vi "velodyne_parse.vi"(5 "Raw LiDAR data":string) -> (1 "Pased LIDAR Data":T1(array[cluster]), 3 "Timestamps":u32[](array[numeric]))   [LabVIEW 2019]
doc: "Parse UDP packet from Velodyne HDL."
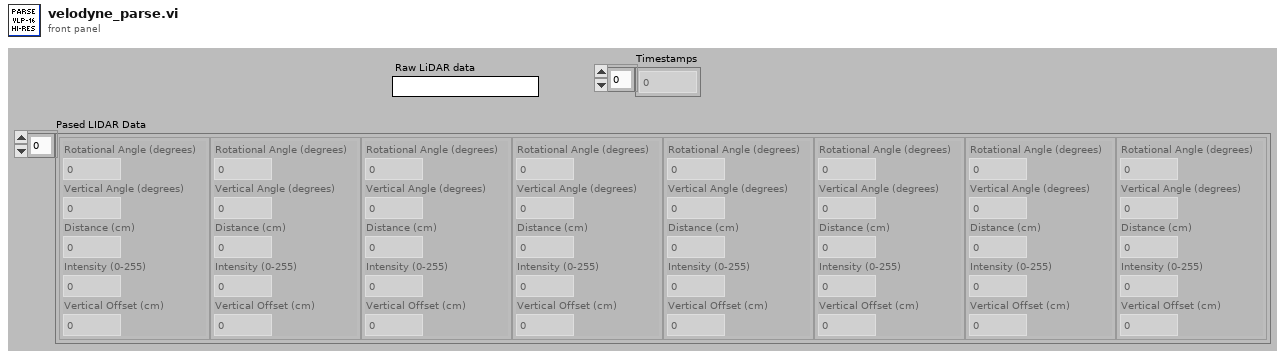
[diagram p1: front panel]
types:
  T1 = cluster{"Rotational Angle (degrees)":dbl, "Vertical Angle (degrees)":dbl, "Distance (cm)":dbl, "Intensity (0-255)":u8, "Vertical Offset (cm)":dbl}[]
  T2 = cluster{"Rotational Angle (degrees)":dbl, "Vertical Angle (degrees)":dbl, "Distance (cm)":dbl, "Intensity (0-255)":u8, "Vertical Offset (cm)":dbl}
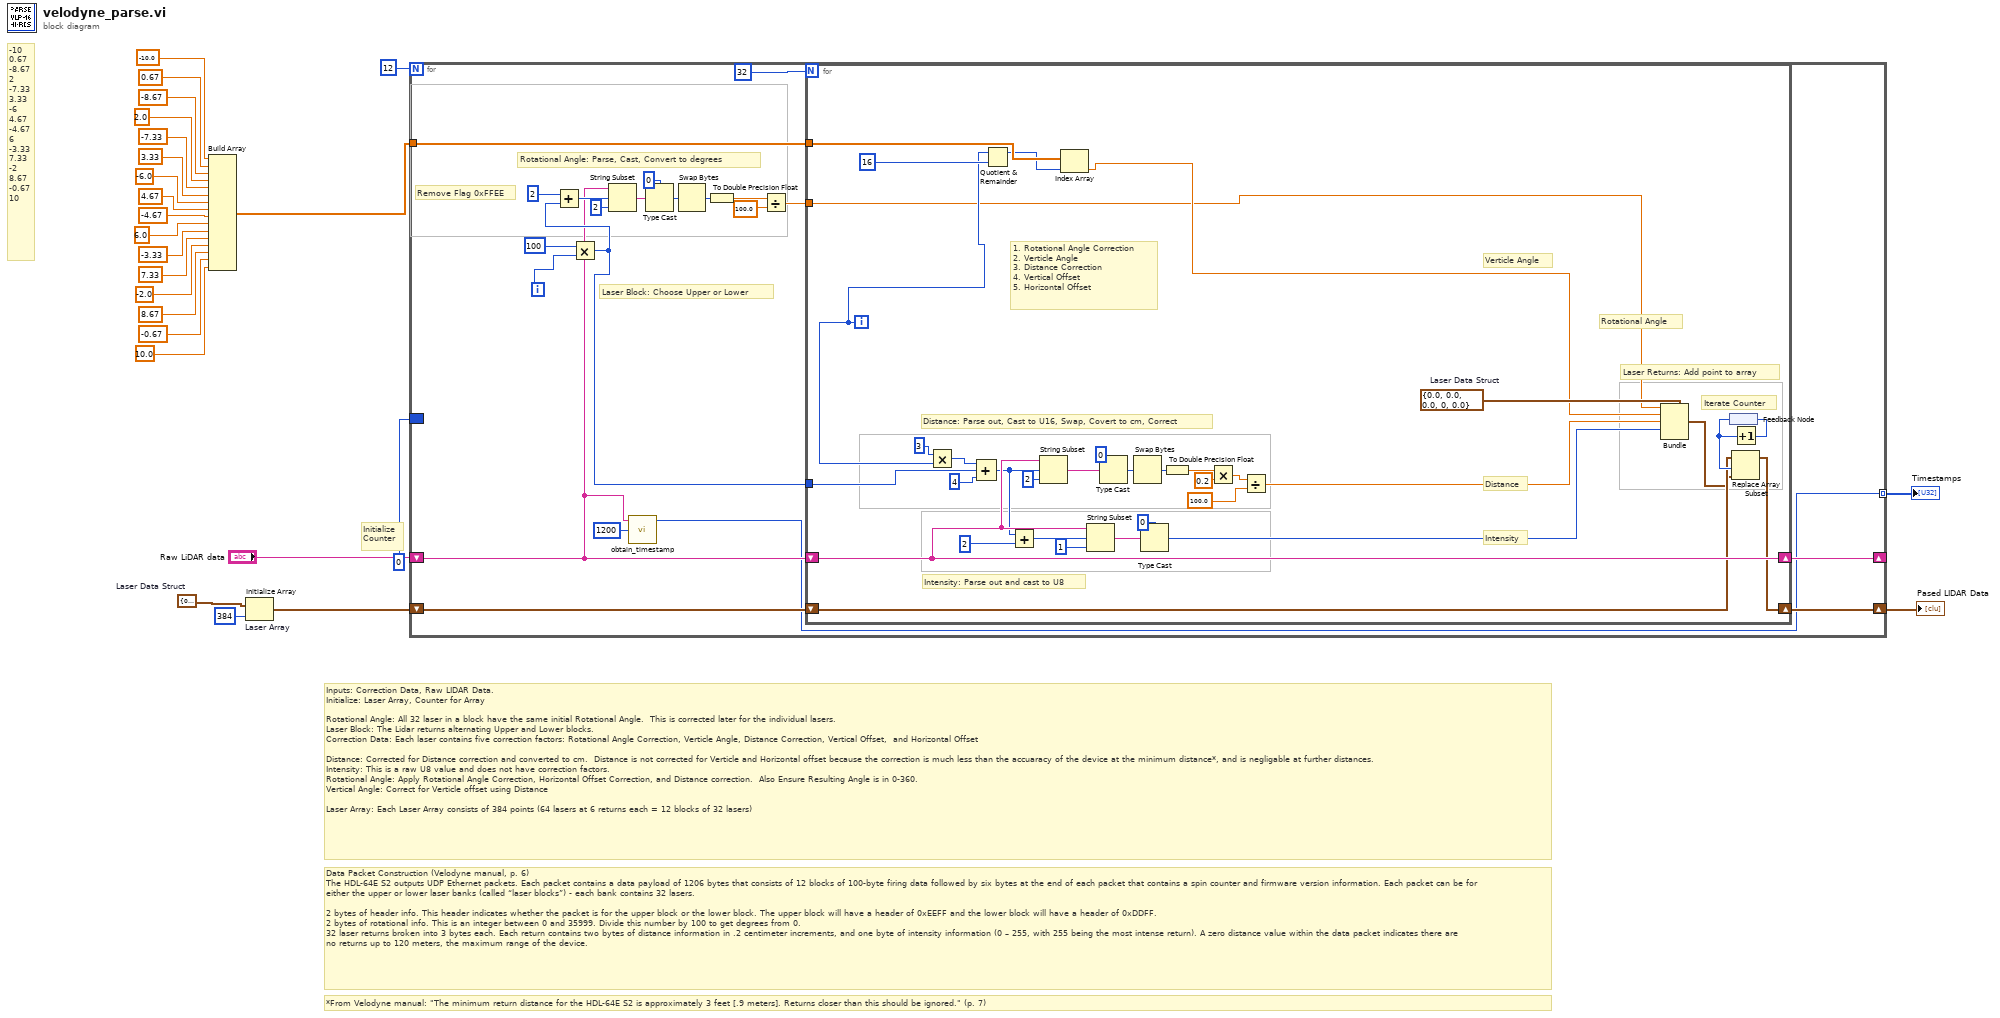
[diagram p0: block diagram]
diagram:
  w24 = T2 {"Rotational Angle (degrees)"=0.0, "Vertical Angle (degrees)"=0.0, "Distance (cm)"=0.0, "Intensity (0-255)"=0, "Vertical Offset (cm)"=0.0}  # Laser Data Struct
  # "-10\n0.67\n-8.67\n2\n-7.33\n3.33\n-6\n4.67\n-4.67\n6\n-3.33\n7.33\n-2\n8.67\n-0.67\n10"
  # "Initialize\nCounter"
  # "Data Packet Construction (Velodyne manual, p. 6)\nThe HDL-64E S2 outputs UDP Ethernet packets. Each packet contains a data payload of 1206 bytes that consists of 12 blocks of 100-byte firing data followed by six bytes at the end of each packet that contains a spin counter and firmware version information. Each packet can be for either the upper or lower laser banks (called “laser blocks”) - each bank contains 32 lasers.\n\n2 bytes of header info. This header indicates whether the packet is for the upper block or the lower block. The upper block will have a header of 0xEEFF and the lower block will have a header of 0xDDFF.\n2 bytes of rotational info. This is an integer between 0 and 35999. Divide this number by 100 to get degrees from 0.\n32 laser returns broken into 3 bytes each. Each return contains two bytes of distance information in .2 centimeter increments, and one byte of intensity information (0 – 255, with 255 being the most intense return). A zero distance value within the data packet indicates there are no returns up to 120 meters, the maximum range of the device."
  # "Inputs: Correction Data, Raw LIDAR Data.\nInitialize: Laser Array, Counter for Array\n\nRotational Angle: All 32 laser in a block have the same initial Rotational Angle.  This is corrected later for the individual lasers.\nLaser Block: The Lidar returns alternating Upper and Lower blocks.\nCorrection Data: Each laser contains five correction factors: Rotational Angle Correction, Verticle Angle, Distance Correction, Vertical Offset,  and Horizontal Offset\n\nDistance: Corrected for Distance correction and converted to cm.  Distance is not corrected for Verticle and Horizontal offset because the correction is much less than the accuaracy of the device at the minimum distance*, and is negligable at further distances.\nIntensity: This is a raw U8 value and does not have correction factors.\nRotational Angle: Apply Rotational Angle Correction, Horizontal Offset Correction, and Distance correction.  Also Ensure Resulting Angle is in 0-360.\nVertical Angle: Correct for Verticle offset using Distance\n\nLaser Array: Each Laser Array consists of 384 points (64 lasers at 6 returns each = 12 blocks of 32 lasers)"
  # "*From Velodyne manual: \"The minimum return distance for the HDL-64E S2 is approximately 3 feet [.9 meters]. Returns closer than this should be ignored.\" (p. 7)"
  n1 = Build Array(-10.0 ("element"), 0.67 ("element"), -8.67 ("element"), 2.0 ("element"), -7.33 ("element"), 3.33 ("element"), -6.0 ("element"), 4.67 ("element"), -4.67 ("element"), 6.0 ("element"), -3.33 ("element"), 7.33 ("element"), -2.0 ("element"), 8.67 ("element"), -0.67 ("element"), 10.0 ("element")) -> (w4:dbl[])
  n2 = Initialize Array "Laser Array"(w24, 384 ("dimension size")) -> (w21:T1)
  n3 = for {
    N: 12 -> [_]
    shift-right: [w41] -> _
    shift-left: "Raw LiDAR data" -> [w27]
    shift-right: [w33] -> w3
    shift-left: w21 -> [w34]
    border: 0 -> [_]
    tunnel: w4 -> [w31]
    tunnel: [w26] -> w1 mode=indexing
    i -> [w32]
    # "Remove Flag 0xFFEE"
    # "Laser Block: Choose Upper or Lower"
    # "Rotational Angle: Parse, Cast, Convert to degrees"
    n4 = Multiply(x=100, y=w32) -> (x*y=w29:i32)
    n5 = Add(x=2, y=w29) -> (x+y=w45:i32)
    n6 = String Subset ("Rotation Angle")(string=w27, offset (0)=w45, length (rest)=2 ("length (rest)")) -> (substring=w38:string)
    n7 = call "obtain_timestamp.vi"("Bit offset (1200)"=1200 ("offset (1200)"), "LiDAR raw data"=w27) -> ("Timestamp (us)"=w26:u32)  [unwired: 3 in]
    n8 = Type Cast(type=u16 0 ("element"), x=w38) -> (*(type *) &x=w39:u16)
    n9 = Swap Bytes(anything=w39) -> (byte swapped=w37:u16)
    n10 = To Double Precision Float(number=w37) -> (double precision float=w36:dbl)
    n11 = Divide(x=w36, y=100.0) -> (x/y=w30:dbl)
    n12 = for {
      N: 32 -> [_]
      shift-right: [w79] -> w41
      shift-left: w27 -> [w79]
      tunnel: w29 -> [w80]
      tunnel: w30 -> [w50]
      shift-right: [w57] -> w33
      shift-left: w34 -> [w58]
      tunnel: w31 -> [w54]
      i -> [w51]
      w60 = T2 {"Rotational Angle (degrees)"=0.0, "Vertical Angle (degrees)"=0.0, "Distance (cm)"=0.0, "Intensity (0-255)"=0, "Vertical Offset (cm)"=0.0}  # Laser Data Struct
      # "Rotational Angle"
      # "Distance"
      # "Intensity"
      # "Verticle Angle"
      # "Iterate Counter"
      # "Laser Returns: Add point to array"
      # "Distance: Parse out, Cast to U16, Swap, Covert to cm, Correct"
      # "Intensity: Parse out and cast to U8"
      # "1. Rotational Angle Correction\n2. Verticle Angle\n3. Distance Correction\n4. Vertical Offset\n5. Horizontal Offset"
      n13 = Multiply(x=3, y=w51) -> (x*y=w75:i32)
      n14 = Compound Arithmetic op=ADD(w75, w80, 4 ("value")) -> (w72:i32)
      n15 = Quotient & Remainder(x=w51, y=16) -> (x-y*floor(x/y)=w52:i32)  [unwired: 1 out]
      n16 = Add(x=w72, y=2) -> (x+y=w71:i32)
      n17 = String Subset ("Distance")(string=w79, offset (0)=w72, length (rest)=2 ("length (rest)")) -> (substring=w66:string)
      n18 = Index Array(array=w54, index=w52) -> (element=w53:dbl)
      n19 = String Subset ("Intensity")(string=w79, offset (0)=w71, length (rest)=1 ("length (rest)")) -> (substring=w69:string)
      n20 = Type Cast(type=u16 0 ("element"), x=w66) -> (*(type *) &x=w67:u16)
      n21 = Swap Bytes(anything=w67) -> (byte swapped=w64:u16)
      n22 = Type Cast(type=u8 0 ("element"), x=w69) -> (*(type *) &x=w59:u8)
      n23 = To Double Precision Float(number=w64) -> (double precision float=w63:dbl)
      n24 = Multiply(x=w63, y=0.2 ("Distance (cm)")) -> (x*y=w49:dbl)
      n25 = Divide(x=w49, y=100.0) -> (x/y=w47:dbl)
      n26 = Bundle(cluster=w60, "Rotational Angle (degrees)"=w50, "Vertical Angle (degrees)"=w53, "Distance (cm)"=w47, "Intensity (0-255)"=w59) -> (w56:T2)  [unwired: 1 in]
      n27 = feedback #1() -> (w62:i32)
      n28 = Replace Array Subset(array=w58, new element=w56, index=w62) -> (w57:T1)
      n29 = Increment(x=w62) -> (x+1=w61:i32)
      n30 = feedback-in #1(w61) -> ()
    }
  }
  "Pased LIDAR Data" <- w3
  "Timestamps" <- w1
